vi "DAQ_2_1.vi"() -> ()   [LabVIEW 2021]
panel:
  in  "Amplitud":dbl(knob) scale=-10.0..10.0
  in  "Stop":bool
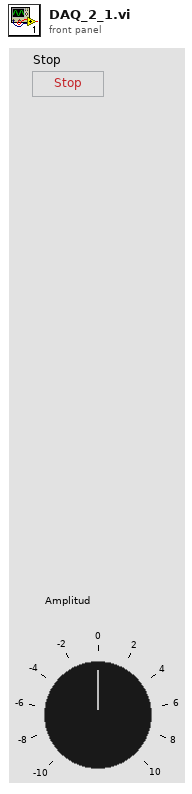
[diagram p1: front panel]
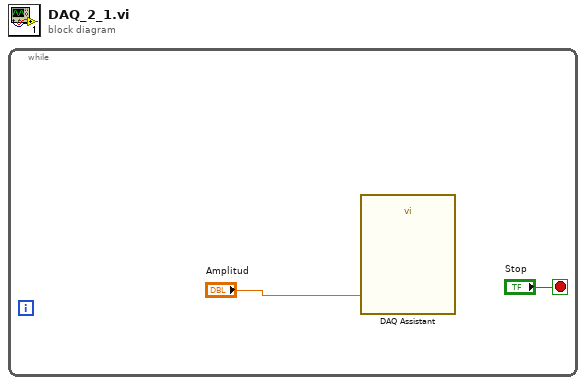
[diagram p0: block diagram]
diagram:
  n1 = while {
    stop <- "Stop" stop-if-true
    n2 = call "DAQ Assistant"("data"="Amplitud") -> ()  [unwired: 17 in, 2 out]
  }
